vi "Parse Response.vi"(11 "Data Array":u8[](array[numeric]) format="%x") -> (3 "Return":T1)   [LabVIEW 2018]
uses:
  Return_t.ctl
panel:
  out "statusMsg":u16 format="%x"
  out "Msg CRC":u16 format="%x"
  out "Msg Length":u16
  out "Opcode":u8 format="%x"
  # "Parse Response"
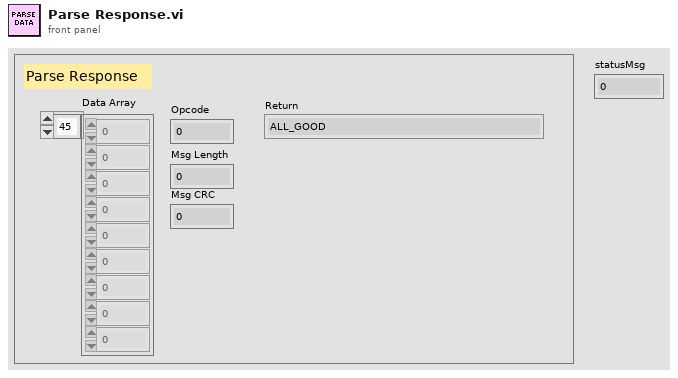
[diagram p1: front panel]
types:
  T1 = typedef "Return_t.ctl" = enum16{"ALL_GOOD", "ERROR_COMMAND_RESPONSE_TIMEOUT", "ERROR_CORRUPT_RESPONSE", "ERROR_WRONG_OPCODE_RESPONSE", "ERROR_UNKNOWN_OPCODE", "RESPONSE_IS_TEMPERATURE", "RESPONSE_IS_KEEPALIVE", "RESPONSE_IS_TEMPTHROTTLE", "RESPONSE_IS_TAGFOUND", "RESPONSE_IS_NOTAGFOUND", "RESPONSE_IS_UNKNOWN", "RESPONSE_SUCCESS", "RESPONSE_FAIL"}
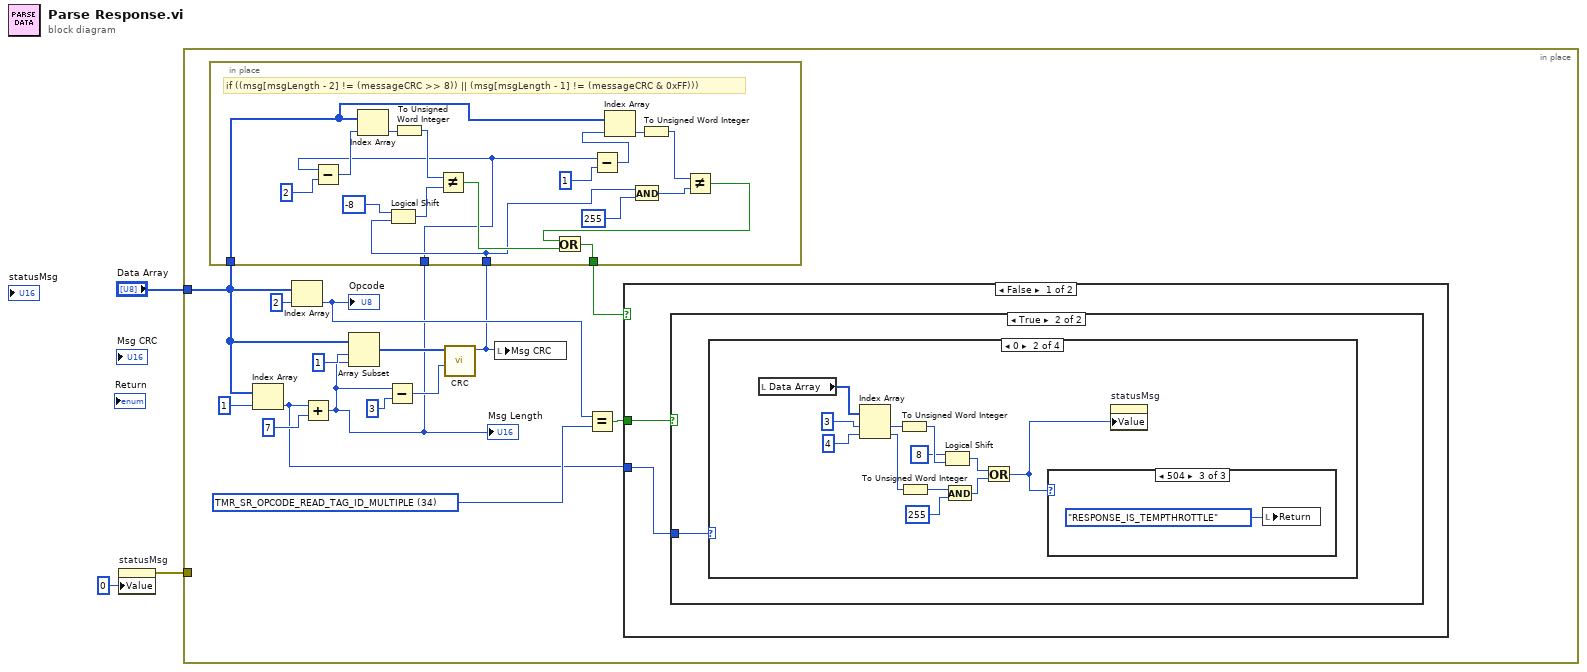
[diagram p0: block diagram]
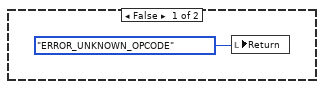
[diagram p2: hidden frame]
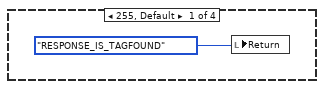
[diagram p3: hidden frame]
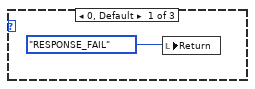
[diagram p4: hidden frame]
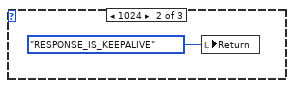
[diagram p5: hidden frame]
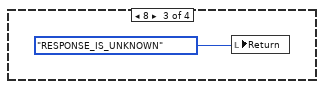
[diagram p6: hidden frame]
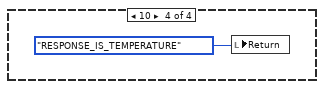
[diagram p7: hidden frame]
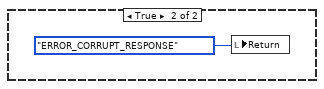
[diagram p8: hidden frame]
diagram:
  n1 = property on="statusMsg" class="DigNum (strict)"("Value"=u16 0 ("statusMsg")) -> (error out=w1:errorcluster)  [unwired: 2 in, 1 out]
  n2 = in-place {
    in-place-border: "Data Array" -> [w9]
    in-place-border: w1 -> [_]
    w13 = u16 34 items=["TMR_SR_OPCODE_VERSION"=3, "TMR_SR_OPCODE_SET_BAUD_RATE"=6, "TMR_SR_OPCODE_READ_TAG_ID_SINGLE"=33, "TMR_SR_OPCODE_READ_TAG_ID_MULTIPLE"=34, "TMR_SR_OPCODE_WRITE_TAG_ID"=35, "TMR_SR_OPCODE_WRITE_TAG_DATA"=36, "TMR_SR_OPCODE_KILL_TAG"=38, "TMR_SR_OPCODE_READ_TAG_DATA"=40, "TMR_SR_OPCODE_CLEAR_TAG_ID_BUFFER"=42, "TMR_SR_OPCODE_MULTI_PROTOCOL_TAG_OP"=47, "TMR_SR_OPCODE_GET_READ_TX_POWER"=98, "TMR_SR_OPCODE_GET_WRITE_TX_POWER"=100, "TMR_SR_OPCODE_GET_POWER_MODE"=104, "TMR_SR_OPCODE_GET_READER_OPTIONAL_PARAMS"=106, "TMR_SR_OPCODE_GET_PROTOCOL_PARAM"=107, "TMR_SR_OPCODE_SET_ANTENNA_PORT"=145, "TMR_SR_OPCODE_SET_TAG_PROTOCOL"=147, "TMR_SR_OPCODE_SET_READ_TX_POWER"=146, "TMR_SR_OPCODE_SET_WRITE_TX_POWER"=148, "TMR_SR_OPCODE_SET_REGION"=151, "TMR_SR_OPCODE_SET_READER_OPTIONAL_PARAMS"=154, "TMR_SR_OPCODE_SET_PROTOCOL_PARAM"=155] ("Opcode Constant")
    n3 = Index Array(array=w9, index=1) -> (element=w10:u8)
    n4 = Index Array(array=w9, index=2) -> (element=w14:u8)
    "Opcode" <- w14
    n5 = Add(x=w10, y=u8 7) -> (x+y=w4:u8)
    "Msg Length" <- w4
    n6 = Array Subset(array=w9, index=1, length=w4) -> (w11:u8[])
    n7 = Subtract(x=w4, y=u8 3) -> (x-y=w7:u8)
    n8 = call "CRC.vi"("Len"=w7, "u8Buf"=w11) -> ("CRC"=w5:u16)  [unwired: 9 in]
    n9 = in-place {
      in-place-border: w9 -> [w26]
      in-place-border: [w21] -> w8
      in-place-border: w5 -> [w20]
      in-place-border: w4 -> [w19]
      # "if ((msg[msgLength - 2] != (messageCRC >> 8)) || (msg[msgLength - 1] != (messageCRC & 0xFF)))"
      n10 = Subtract(x=w19, y=u16 2) -> (x-y=w36:u16)
      n11 = Index Array(array=w26, index=w36) -> (element=w33:u8)
      n12 = Logical Shift(y=i16 -8, x=w20) -> (x << y=w31:u16)
      n13 = To Unsigned Word Integer(number=w33) -> (unsigned 16bit integer=w32:u16)
      n14 = Not Equal?(x=w32, y=w31) -> (x != y?=w23:bool)
      n15 = Subtract(x=w19, y=u16 1) -> (x-y=w27:u16)
      n16 = Index Array(array=w26, index=w27) -> (element=w29:u8)
      n17 = And(x=w20, y=u16 255) -> (x .and. y?=w24:u16)
      n18 = To Unsigned Word Integer(number=w29) -> (unsigned 16bit integer=w30:u16)
      n19 = Not Equal?(x=w30, y=w24) -> (x != y?=w22:bool)
      n20 = Or(x=w22, y=w23) -> (x .or. y?=w21:bool)
    }
    n21 = local write "Msg CRC"(w5) -> ()
    n22 = Equal?(x=w14, y=w13) -> (x = y?=w12:bool)
    n23 = case shown="False" w8 {
      tunnel: w12 -> [w38 _]
      tunnel: w10 -> [w37 _]
      frame False {
        n24 = case shown="True" w38 {
          tunnel: w37 -> [_ w40]
          frame False {
            n25 = local write "Return"(Return_t."ERROR_UNKNOWN_OPCODE" ("Return")) -> ()
          }
          frame True {
            n26 = case shown="0" w40 {
              frame 255, Default {
                n27 = local write "Return"(Return_t."RESPONSE_IS_TAGFOUND" ("Return")) -> ()
              }
              frame 0 {
                n28 = local read "Data Array"() -> (w53:u8[])
                n29 = Index Array(array=w53, index #1=3 ("y"), index #2=4 ("y")) -> (element #1=w52:u8, element #2=w45:u8)
                n30 = To Unsigned Word Integer(number=w52) -> (unsigned 16bit integer=w51:u16)
                n31 = To Unsigned Word Integer(number=w45) -> (unsigned 16bit integer=w44:u16)
                n32 = Logical Shift(y=i16 8, x=w51) -> (x << y=w50:u16)
                n33 = And(x=w44, y=u16 255) -> (x .and. y?=w42:u16)
                n34 = Or(x=w50, y=w42) -> (x .or. y?=w49:u16)
                n35 = case shown="504" w49 {
                  frame 0, Default {
                    n36 = local write "Return"(Return_t."RESPONSE_FAIL" ("Return")) -> ()
                  }
                  frame 1024 {
                    n37 = local write "Return"(Return_t."RESPONSE_IS_KEEPALIVE" ("Return")) -> ()
                  }
                  frame 1284 {
                    n38 = local write "Return"(Return_t."RESPONSE_IS_TEMPTHROTTLE" ("Return")) -> ()
                  }
                }
                n39 = property on="statusMsg" class="DigNum (strict)"("Value"=w49) -> ()  [unwired: 2 in, 2 out]
              }
              frame 8 {
                n40 = local write "Return"(Return_t."RESPONSE_IS_UNKNOWN" ("Return")) -> ()
              }
              frame 10 {
                n41 = local write "Return"(Return_t."RESPONSE_IS_TEMPERATURE" ("Return")) -> ()
              }
            }
          }
        }
      }
      frame True {
        n42 = local write "Return"(Return_t."ERROR_CORRUPT_RESPONSE" ("Return")) -> ()
      }
    }
  }
